vi "LV GET REGISTER.vi"(9 "Board Handle In":T1, 11 "Register Name":string) -> (0 "NI Error Code":i32, 1 "Board Handle Out":T1, 3 "Register Value":u32)   [LabVIEW 2021, in "SciSDK_Labview.lvlib"]
uses:
  SciSDK_Labview.lvlib
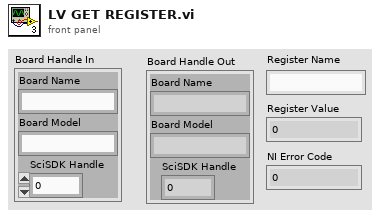
[diagram p1: front panel]
types:
  T1 = cluster{"Board Name":string, "Board Model":string, "SciSDK Handle":u64}
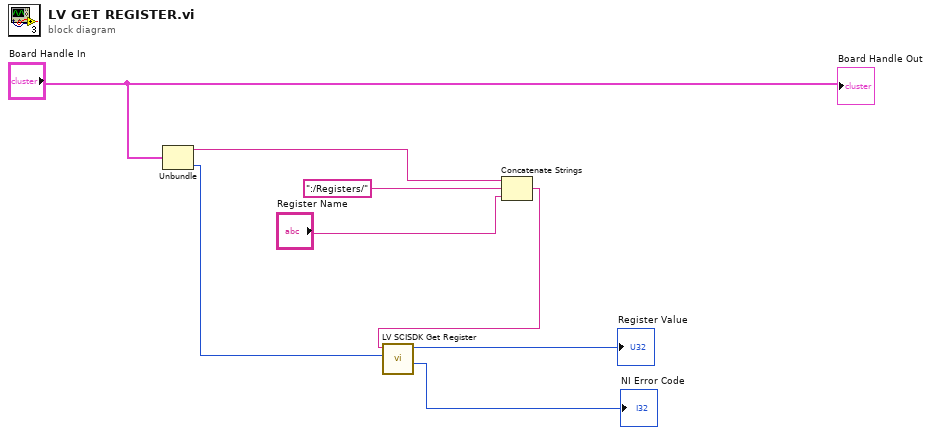
[diagram p0: block diagram]
diagram:
  n1 = Unbundle("Board Handle In") -> ("Board Name"=w7:string, "SciSDK Handle"=w2:u64)  [unwired: 1 out]
  n2 = Concatenate Strings(w7, ":/Registers/" ("string"), "Register Name") -> (w4:string)
  n3 = call "LV SCISDK Get Register.vi"("handle"=w2, "Path"=w4) -> ("function return"=→"NI Error Code":i32, "value"=→"Register Value":u32)  [unwired: 6 in, 2 out]
  "Board Handle Out" <- "Board Handle In"
